vi "Floating Intake Read.vi"(7 "Description":string, 8 "Command Info In":T1, 11 "Setpoint":dbl) -> (0 "Command Info Out":T1, 2 "Current":dbl)   [LabVIEW 2018]
doc: "This template is useful for immediate subsystem actions that do not need deadband filtering\n\nBe sure to right-click and select New from Template and save with a new command name."
uses:
  <vilib>/Rock Robotics/WPI/Framework/Command Status Info.ctl
  <vilib>/Rock Robotics/WPI/Framework/Completion Status.ctl
  <vilib>/Rock Robotics/WPI/Framework/Completion Notifier.ctl
  Implementation/Floating Intake Setpoints.ctl
  Implementation/Floating Intake Operations.ctl
  <vilib>/Rock Robotics/Network Tables/NT Read Number.vi
  <vilib>/Rock Robotics/Network Tables/NT Write Number.vi
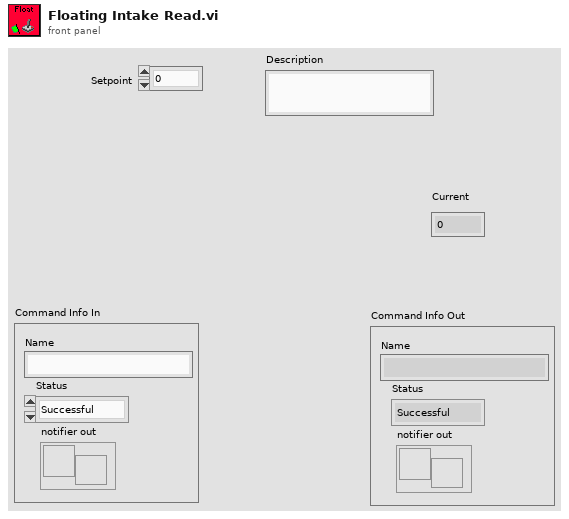
[diagram p1: front panel]
types:
  T1 = typedef "Command Status Info.ctl" = cluster{"Name":string, "Status":T2, "notifier out":T3}
  T2 = typedef "Completion Status.ctl" = enum16{"Successful", "Aborted", "Incomplete"}
  T3 = typedef "Completion Notifier.ctl" = refnum<notifier>
  T4 = typedef "Floating Intake Setpoints.ctl" = cluster{"Operation":T5, "Setpoint":dbl, "Duration":dbl, "extend":bool}
  T5 = typedef "Floating Intake Operations.ctl" = enum16{"Reserve", "Read Current", "Immediate", "Duration"}
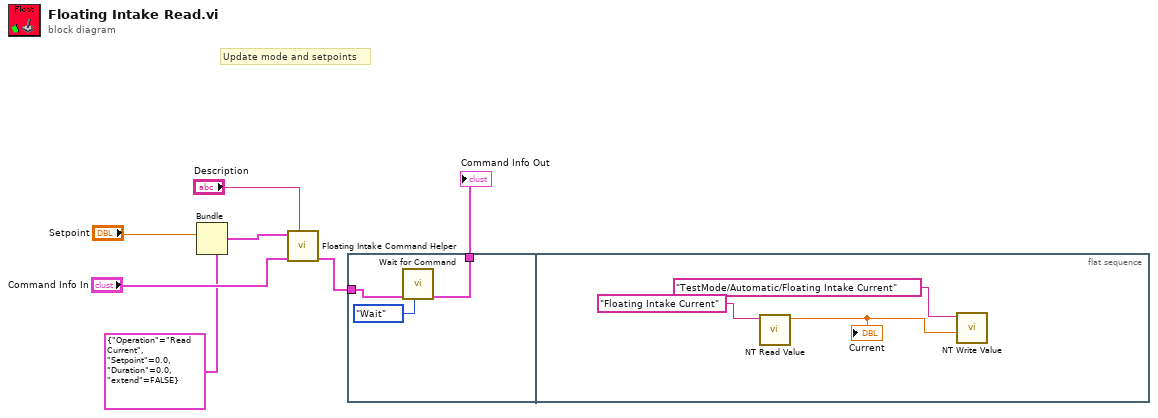
[diagram p0: block diagram]
diagram:
  # "Update mode and setpoints"
  n1 = Bundle(cluster=T4 {"Operation"=enum."Read Current", "Setpoint"=0.0, "Duration"=0.0, "extend"=FALSE} ("SubSystem Data"), "Setpoint"="Setpoint") -> (w3:T4)  [unwired: 3 in]
  n2 = call "Floating Intake Command Helper.vi"("Description"="Description", "Command Info In"="Command Info In", "SubSystem Data"=w3) -> ("Command Info Out"=w2:T1)  [unwired: 6 in, 2 out]
  n3 = flat-sequence {
    tunnel: w2 -> [w10]
    tunnel: [w9] -> w1
    frame #0 {
      n4 = call <vilib>:"Wait for Command.vi"("Synchronication"=enum16{"Start", "Wait"}."Wait", "Command Info in"=w10) -> ("Command Info out"=w9:T1)  [unwired: 9 in]
    }
    frame #1 {
      n5 = call-poly <vilib>:"NT Read Value.vi"("Name"="Floating Intake Current") -> ("Numeric"=w11:dbl)  [unwired: 9 in, 1 out]
      "Current" <- w11
      n6 = call-poly <vilib>:"NT Write Value.vi"("Numeric"=w11, "Name"="TestMode/Automatic/Floating Intake Current") -> ()  [unwired: 9 in, 1 out]
    }
  }
  "Command Info Out" <- w1
